vi "DistanceToLine.vi"(10 "Irons direct vector out":T1, 11 "Robot UTM Location":T2 {"North" format="%#_10f"; "East" format="%#_8f"}) -> (2 "Distance":dbl)   [LabVIEW 2011]
doc: "Takes in a line from original robot location to the goal and calculates the distance between the robot and the line."
uses:
  2 Typedefs/UTM Location.ctl
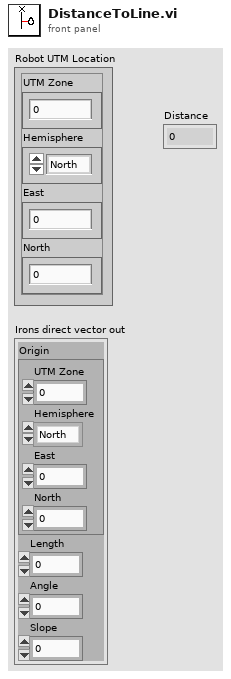
[diagram p1: front panel]
types:
  T1 = cluster{"Origin":cluster{"UTM Zone":dbl, "Hemisphere":enum16{"North", "South"}, "East":dbl, "North":dbl}, "Length":dbl, "Angle":dbl, "Slope":dbl}
  T2 = typedef "UTM Location.ctl" = cluster{"UTM Zone":dbl, "Hemisphere":enum16{"North", "South"}, "East":dbl, "North":dbl}
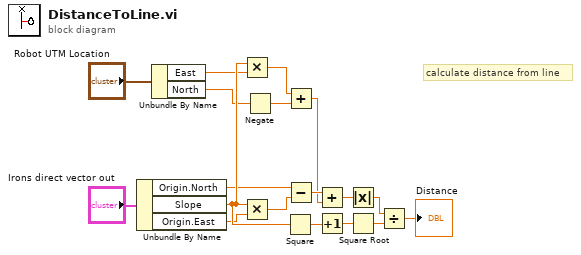
[diagram p0: block diagram]
diagram:
  # "calculate distance from line"
  n1 = Unbundle By Name("Irons direct vector out") -> ("Origin.North"=w1:dbl, "Slope"=w13:dbl, "Origin.East"=w2:dbl)
  n2 = Unbundle By Name("Robot UTM Location") -> ("East"=w4:dbl, "North"=w6:dbl)
  n3 = Multiply(x=w13, y=w4) -> (x*y=w5:dbl)
  n4 = Multiply(x=w13, y=w2) -> (x*y=w3:dbl)
  n5 = Negate(x=w6) -> (-x=w7:dbl)
  n6 = Square(x=w13) -> (x^2=w14:dbl)
  n7 = Add(x=w5, y=w7) -> (x+y=w8:dbl)
  n8 = Subtract(x=w1, y=w3) -> (x-y=w9:dbl)
  n9 = Add(x=w9, y=w8) -> (x+y=w10:dbl)
  n10 = Increment(x=w14) -> (x+1=w15:dbl)
  n11 = Absolute Value(x=w10) -> (abs(x)=w11:dbl)
  n12 = Square Root(x=w15) -> (sqrt(x)=w12:dbl)
  n13 = Divide(x=w11, y=w12) -> (x/y=→"Distance":dbl)
